vi "Tektronix TTR500 Series Thru Between Port 1 and Port 2 Calibration.vi"() -> ()   [LabVIEW 2012]
doc: "This VI performs thru calibration between port 1 and port 2.\n\nFor this VI you must set THRU between Port 1 and Port 2 on instrument."
uses:
  <instrlib>/Tektronix TTR500 Series/Tektronix TTR500 Series.lvlib
panel:
  in  "Reset? (T: Yes)":bool=TRUE
  in  "ID Query? (T: Yes)":bool=TRUE
  in  "VISA resource name":refnum<visa-resource-name>
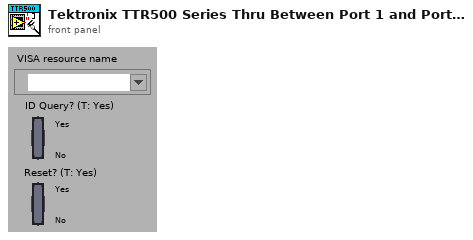
[diagram p1: front panel]
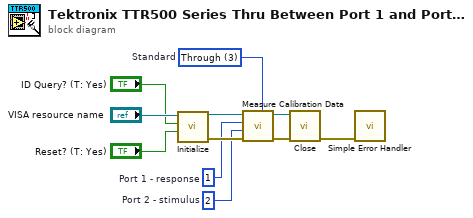
[diagram p0: block diagram]
diagram:
  w1 = u16 3 items=["Open", "Short", "Load", "Through", "Isolation", "Gain Phase Open", "Gain Phase Short", "Gain Phase Load", "Gain Phase Through", "Gain Phase Isolation"]  # Standard
  w5 = 2  # Port 2 - stimulus
  w6 = 1  # Port 1 - response
  n1 = call <instrlib>:"Initialize.vi"("Reset? (T: Yes)"="Reset? (T: Yes)", "ID Query? (T: Yes)"="ID Query? (T: Yes)", "VISA resource name"="VISA resource name") -> ("error out"=w7:errorcluster, "VISA resource name out"=w8:refnum<visa-resource-name>)  [unwired: 6 in, 1 out]
  n2 = call <instrlib>:"Measure Calibration Data.vi"("Standard (0: Open)"=w1, "error in (no error)"=w7, "Port 2 - stimulus (2)"=w5, "Port 1 - response (1)"=w6, "VISA resource name"=w8) -> ("error out"=w2:errorcluster, "VISA resource name out"=w3:refnum<visa-resource-name>)  [unwired: 5 in]
  n3 = call <instrlib>:"Close.vi"("error in (no error)"=w2, "VISA resource name"=w3) -> ("error out"=w4:errorcluster)  [unwired: 9 in]
  n4 = call <vilib>:"Simple Error Handler.vi"("error in (no error)"=w4) -> ()  [unwired: 4 in, 5 out]
